vi "plus-minus.vi"(10 "String 2":string, 11 "String":string) -> (3 "String 3":string)   [LabVIEW 2025]
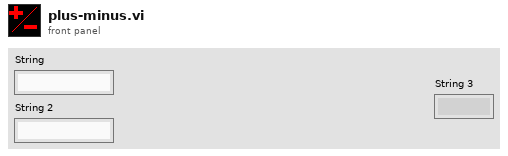
[diagram p1: front panel]
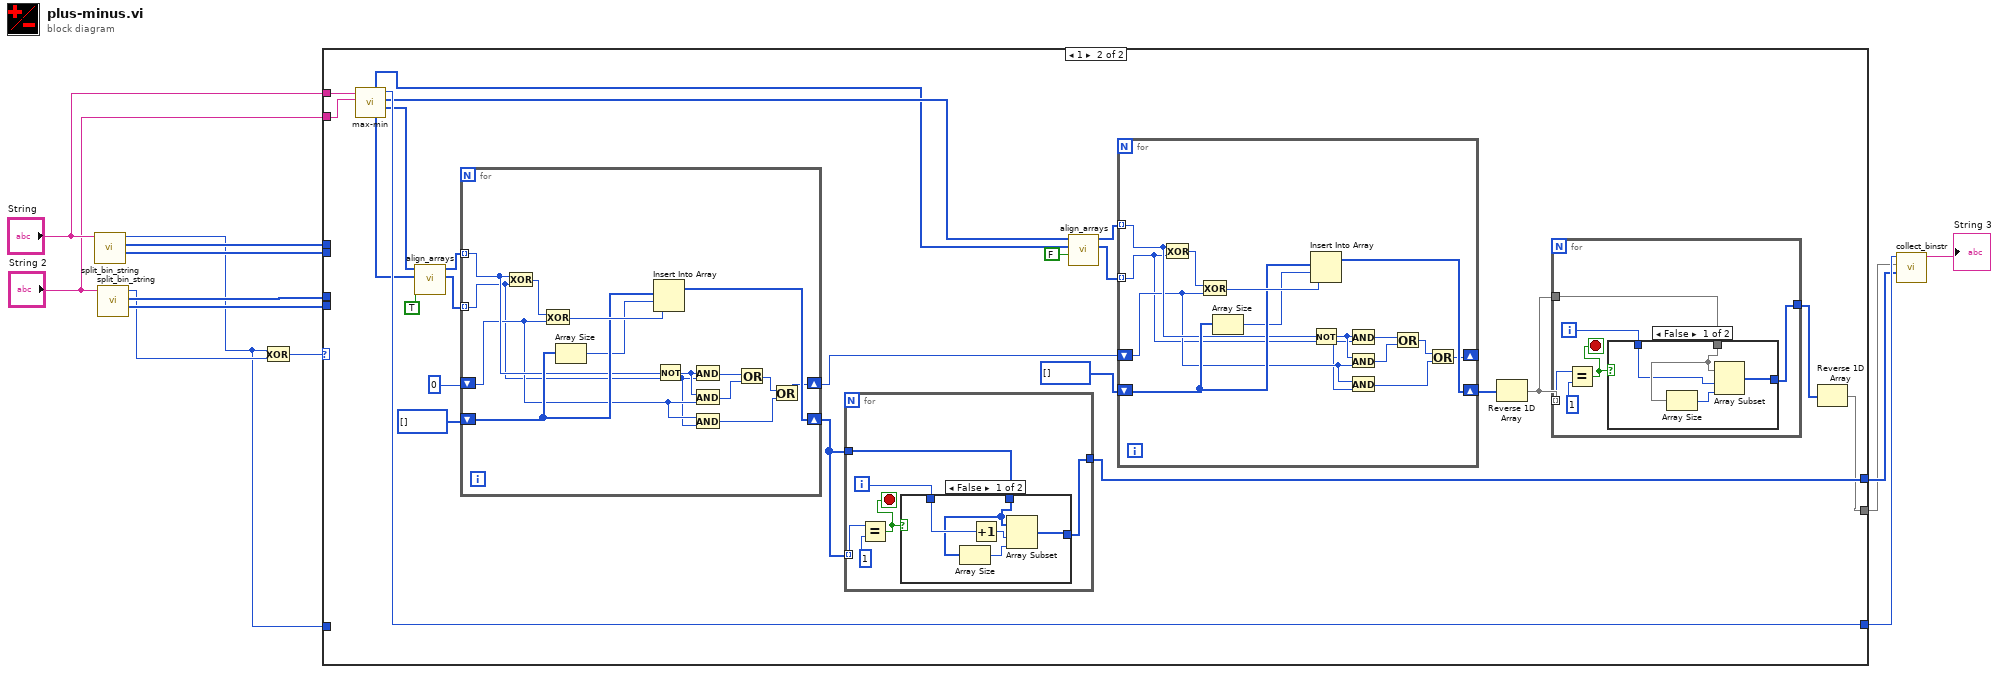
[diagram p0: block diagram]
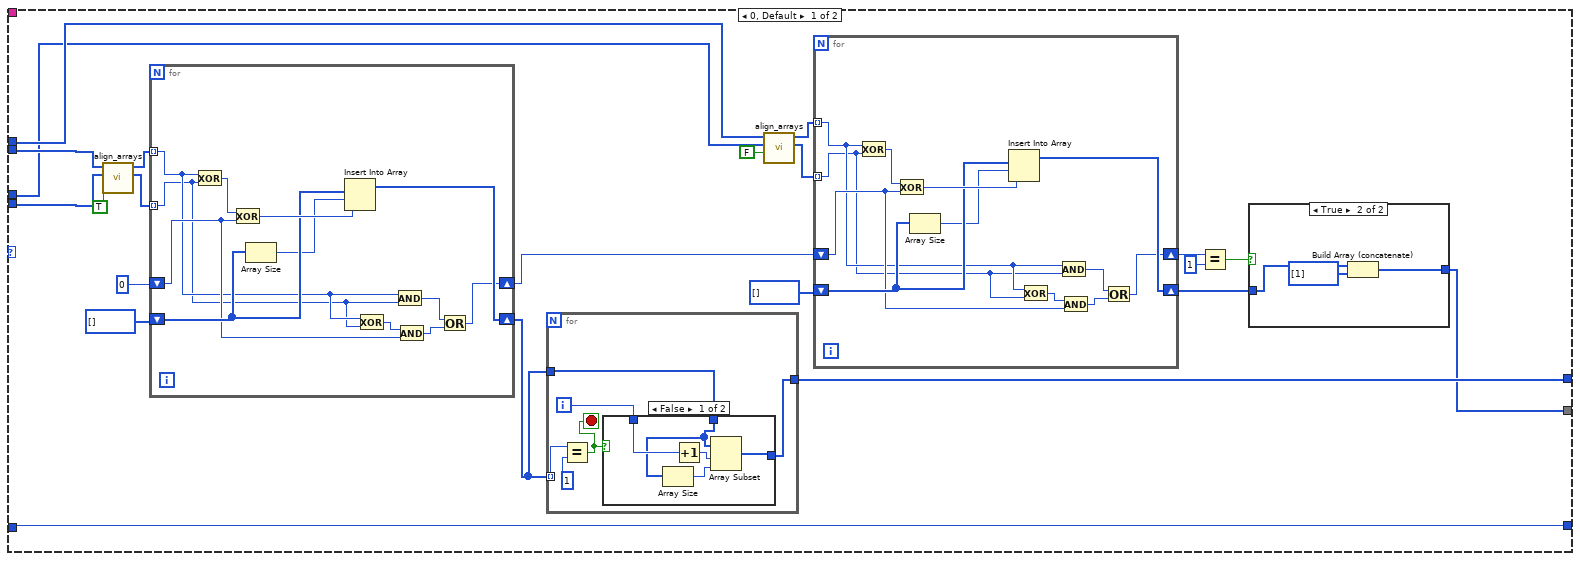
[diagram p2: hidden frame]
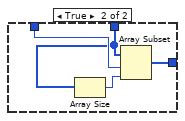
[diagram p4: hidden frame]
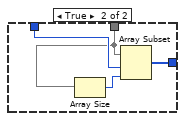
[diagram p5: hidden frame]
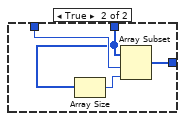
[diagram p6: hidden frame]
diagram:
  n1 = call "split_bin_string.vi"("String"="String") -> ("Fraction"=w12:u8[], "Integer"=w10:u8[], "Sign"=w6:u8)  [unwired: 8 in]
  n2 = call "split_bin_string.vi"("String"="String 2") -> ("Fraction"=w11:u8[], "Integer"=w9:u8[], "Sign"=w8:u8)  [unwired: 8 in]
  n3 = Exclusive Or(1:w8, 2:w6) -> (0:w7:u8)
  n4 = case shown="1" w7 {
    tunnel: w12 -> [w20 _]
    tunnel: w11 -> [w18 _]
    tunnel: [w17 w86] -> w4
    tunnel: w10 -> [w21 _]
    tunnel: w9 -> [w19 _]
    tunnel: [w16 w79] -> w1
    tunnel: w6 -> [w15 _]
    tunnel: [w15 w90] -> w5
    tunnel: "String" -> [_ w92]
    tunnel: "String 2" -> [_ w91]
    frame 0, Default {
      n5 = call "align_arrays.vi"("IS_FRACTION"=TRUE, "Array 2"=w18, "Array"=w20) -> ("Array 4"=w34:u8[], "Array 3"=w33:u8[])  [unwired: 7 in]
      n6 = for {
        tunnel: w33 -> [w68] mode=indexing
        tunnel: w34 -> [w67] mode=indexing
        shift-right: [w69] -> w30
        shift-left: u8 0 -> [w73]
        shift-right: [w74] -> w14
        shift-left: u8[] [] -> [w76]
        n7 = Exclusive Or(1:w67, 2:w68) -> (0:w78:u8)
        n8 = Exclusive Or(1:w73, 2:w78) -> (0:w77:u8)
        n9 = Array Size(array=w76) -> (size(s)=w75:i32)
        n10 = Insert Into Array(array=w76, index=w75, new element=w77) -> (w74:u8[])
        n11 = Exclusive Or(1:w67, 2:w68) -> (0:w72:u8)
        n12 = And(x=w68, y=w67) -> (x .and. y?=w70:u8)
        n13 = And(x=w72, y=w73) -> (x .and. y?=w71:u8)
        n14 = Or(x=w70, y=w71) -> (x .or. y?=w69:u8)
      }
      n15 = for {
        tunnel: w14 -> [w57] mode=indexing
        tunnel: w14 -> [w53]
        tunnel: [w52] -> w17
        i -> [w54]
        stop <- w55 stop-if-true
        n16 = Equal?(x=w57, y=u8 1) -> (x = y?=w55:bool)
        n17 = case shown="False" w55 {
          tunnel: w54 -> [w61 w66]
          tunnel: w53 -> [w60 w65]
          tunnel: [w58 w63] -> w52
          frame False {
            n18 = Array Size(array=w60) -> (size(s)=w59:i32)
            n19 = Increment(x=w61) -> (x+1=w62:i32)
            n20 = Array Subset(array=w60, index=w62, length=w59) -> (w58:u8[])
          }
          frame True {
            n21 = Array Size(array=w65) -> (size(s)=w64:i32)
            n22 = Array Subset(array=w65, index=w66, length=w64) -> (w63:u8[])
          }
        }
      }
      n23 = call "align_arrays.vi"("IS_FRACTION"=FALSE, "Array 2"=w19, "Array"=w21) -> ("Array 4"=w26:u8[], "Array 3"=w27:u8[])  [unwired: 7 in]
      n24 = for {
        tunnel: w27 -> [w41] mode=indexing
        tunnel: w26 -> [w40] mode=indexing
        shift-right: [w42] -> w25
        shift-left: w30 -> [w46]
        shift-right: [w47] -> w22
        shift-left: u8[] [] -> [w49]
        n25 = Exclusive Or(1:w40, 2:w41) -> (0:w51:u8)
        n26 = Exclusive Or(1:w46, 2:w51) -> (0:w50:u8)
        n27 = Array Size(array=w49) -> (size(s)=w48:i32)
        n28 = Insert Into Array(array=w49, index=w48, new element=w50) -> (w47:u8[])
        n29 = Exclusive Or(1:w40, 2:w41) -> (0:w45:u8)
        n30 = And(x=w41, y=w40) -> (x .and. y?=w43:u8)
        n31 = And(x=w45, y=w46) -> (x .and. y?=w44:u8)
        n32 = Or(x=w43, y=w44) -> (x .or. y?=w42:u8)
      }
      n33 = Equal?(x=w25, y=u8 1) -> (x = y?=w23:bool)
      n34 = case shown="True" w23 {
        tunnel: w22 -> [w36 w39]
        tunnel: [w36 w38] -> w16
        frame False {
        }
        frame True {
          n35 = Build Array (concatenate)(w39, u8[] [1] ("array")) -> (w38:u8[])
        }
      }
    }
    frame 1 {
      n36 = call "max-min.vi"("String 2"=w91, "String"=w92) -> ("Fraction"=w89:u8[], "Integer"=w87:u8[], "Sign"=w90:u8, "Fraction 2"=w88:u8[], "Integer 2"=w84:u8[])  [unwired: 4 in, 1 out]
      n37 = call "align_arrays.vi"("IS_FRACTION"=TRUE, "Array 2"=w88, "Array"=w89) -> ("Array 4"=w100:u8[], "Array 3"=w99:u8[])  [unwired: 7 in]
      n38 = for {
        tunnel: w99 -> [w152] mode=indexing
        tunnel: w100 -> [w150] mode=indexing
        shift-right: [w145] -> w93
        shift-left: u8 0 -> [w151]
        shift-right: [w154] -> w85
        shift-left: u8[] [] -> [w156]
        n39 = Exclusive Or(1:w150, 2:w152) -> (0:w158:u8)
        n40 = Exclusive Or(1:w151, 2:w158) -> (0:w157:u8)
        n41 = Array Size(array=w156) -> (size(s)=w155:i32)
        n42 = Insert Into Array(array=w156, index=w155, new element=w157) -> (w154:u8[])
        n43 = Not(x=w152) -> (.not. x?=w153:u8)
        n44 = And(x=w153, y=w150) -> (x .and. y?=w149:u8)
        n45 = And(x=w153, y=w151) -> (x .and. y?=w148:u8)
        n46 = And(x=w151, y=w150) -> (x .and. y?=w146:u8)
        n47 = Or(x=w149, y=w148) -> (x .or. y?=w147:u8)
        n48 = Or(x=w147, y=w146) -> (x .or. y?=w145:u8)
      }
      n49 = for {
        tunnel: w85 -> [w121] mode=indexing
        tunnel: w85 -> [w117]
        tunnel: [w116] -> w86
        i -> [w118]
        stop <- w119 stop-if-true
        n50 = Equal?(x=w121, y=u8 1) -> (x = y?=w119:bool)
        n51 = case shown="False" w119 {
          tunnel: w118 -> [w125 w130]
          tunnel: w117 -> [w124 w129]
          tunnel: [w122 w127] -> w116
          frame False {
            n52 = Array Size(array=w124) -> (size(s)=w123:i32)
            n53 = Increment(x=w125) -> (x+1=w126:i32)
            n54 = Array Subset(array=w124, index=w126, length=w123) -> (w122:u8[])
          }
          frame True {
            n55 = Array Size(array=w129) -> (size(s)=w128:i32)
            n56 = Array Subset(array=w129, index=w130, length=w128) -> (w127:u8[])
          }
        }
      }
      n57 = call "align_arrays.vi"("IS_FRACTION"=FALSE, "Array 2"=w84, "Array"=w87) -> ("Array 4"=w94:u8[], "Array 3"=w95:u8[])  [unwired: 7 in]
      n58 = for {
        tunnel: w95 -> [w134] mode=indexing
        tunnel: w94 -> [w132] mode=indexing
        shift-right: [w131] -> _
        shift-left: w93 -> [w133]
        shift-right: [w140] -> w82
        shift-left: u8[] [] -> [w142]
        n59 = Exclusive Or(1:w132, 2:w134) -> (0:w144:u8)
        n60 = Exclusive Or(1:w133, 2:w144) -> (0:w143:u8)
        n61 = Array Size(array=w142) -> (size(s)=w141:i32)
        n62 = Insert Into Array(array=w142, index=w141, new element=w143) -> (w140:u8[])
        n63 = Not(x=w134) -> (.not. x?=w139:u8)
        n64 = And(x=w139, y=w132) -> (x .and. y?=w138:u8)
        n65 = And(x=w139, y=w133) -> (x .and. y?=w137:u8)
        n66 = And(x=w133, y=w132) -> (x .and. y?=w135:u8)
        n67 = Or(x=w138, y=w137) -> (x .or. y?=w136:u8)
        n68 = Or(x=w136, y=w135) -> (x .or. y?=w131:u8)
      }
      n69 = Reverse 1D Array(array=w82) -> (reversed array=w81:u8[])
      n70 = for {
        tunnel: w81 -> [w107] mode=indexing
        tunnel: w81 -> [w103]
        tunnel: [w102] -> w80
        i -> [w104]
        stop <- w105 stop-if-true
        n71 = Equal?(x=w107, y=u8 1) -> (x = y?=w105:bool)
        n72 = case shown="False" w105 {
          tunnel: w104 -> [w108 w115]
          tunnel: w103 -> [w111 w114]
          tunnel: [w109 w112] -> w102
          frame False {
            n73 = Array Size(array=w111) -> (size(s)=w110:i32)
            n74 = Array Subset(array=w111, index=w108, length=w110) -> (w109:u8[])
          }
          frame True {
            n75 = Array Size(array=w114) -> (size(s)=w113:i32)
            n76 = Array Subset(array=w114, index=w115, length=w113) -> (w112:u8[])
          }
        }
      }
      n77 = Reverse 1D Array(array=w80) -> (reversed array=w79:u8[])
    }
  }
  n78 = call "collect_binstr.vi"("Fraction"=w4, "Integer"=w1, "Sign"=w5) -> ("String"=→"String 3":string)  [unwired: 8 in]
